vi "Init.vi"(8 "error in (no error)":errorcluster, 10 "Address":string, 11 "KIM101.lvlib:KIM101.lvclass":refnum<class "KIM101.lvclass">) -> (0 "error out":errorcluster, 3 "KIM101.lvlib:KIM101.lvclass":refnum<class "KIM101.lvclass">)   [LabVIEW 2023, in "KIM101.lvlib" / "KIM101.lvclass"]
uses:
  KIM101.lvclass
  C:/Program Files/National Instruments/LabVIEW 2023/vi.lib/ActorFramework/Actor/Actor.lvclass
  UIs/TranslationStage_UI/TranslationStage_UI/BPC_Voltages.ctl
  <vilib>/ActorFramework/Message Enqueuer/Message Enqueuer.lvclass
  typedefs/instrumentType.ctl
  KIM101.lvclass/KIM101.ctl
  <vilib>/ActorFramework/Actor/Actor.lvclass/Actor.ctl
  <vilib>/ActorFramework/Message Enqueuer/Message Enqueuer.lvclass/Message Enqueuer.ctl
  Interfaces/InitDeinitInterface/InitDeinitComm Messages/InitDone Msg/InitDone Msg.lvclass/InitDone Msg.ctl
  <vilib>/ActorFramework/Message Enqueuer/Init from Existing Queue.vi
  <vilib>/ActorFramework/Message Enqueuer/Enqueue.vi
  Interfaces/InitDeinitInterface/InitDeinitComm Messages/InitDone Msg/InitDone Msg.lvclass
  C:/Program Files/National Instruments/LabVIEW 2023/vi.lib/ActorFramework/Message/Message.lvclass
  <vilib>/ActorFramework/Message Priority Queue/Priority Enqueue.vi
  C:/Users/quantum/Documents/LVDAQ/UIs/TranslationStage_UI/Thorlabs.MotionControl.KCube.InertialMotorCLI.dll
  UIs/TranslationStage_UI/Thorlabs.MotionControl.KCube.InertialMotorCLI.dll
  KIM101.lvlib
  typedefs/typedefs.lvlib
  <vilib>/ActorFramework/Actor/Actor.lvclass
  C:/Users/quantum/Documents/LVDAQ/UIs/TranslationStage_UI/Thorlabs.MotionControl.Controls.dll
  UIs/TranslationStage_UI/Thorlabs.MotionControl.Controls.dll
panel:
  out "output cluster":T3
  out "KIM Enqueuer":refnum<class "Message Enqueuer.lvclass">
  in  "KIM Positions":T1
  in  "KCubeInertialMotorControl":refnum<k24>(container)
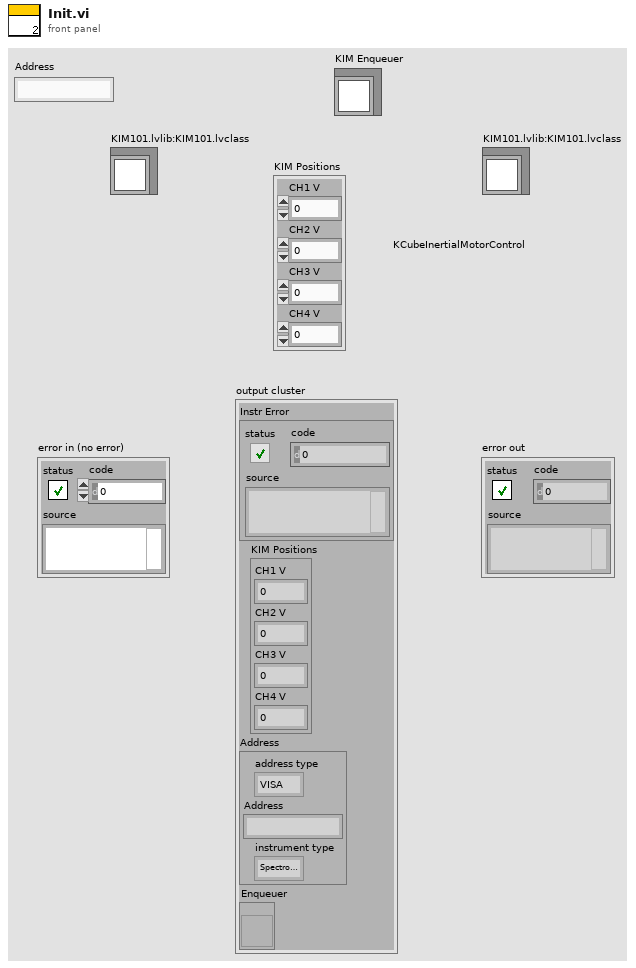
[diagram p1: front panel]
types:
  T1 = typedef "typedefs.lvlib/BPC_Voltages.ctl" = cluster{"CH1 V":i32, "CH2 V":i32, "CH3 V":i32, "CH4 V":i32}
  T2 = typedef "typedefs.lvlib/instrumentType.ctl" = enum16{"Spectrometer", "Camera", "Stepper", "Piezo"}
  T3 = cluster{"Instr Error":errorcluster, "KIM Positions":T1, "Address":cluster{"address type":enum16{"VISA", "Index"}, "Address":string, "instrument type":T2}, "Enqueuer":refnum<vi>}
  T4 = cluster{"JogAcceleration":i32, "JogStepFwd":i32, "JogMode":i32, "JogRate":i32, "JogStepRev":i32}
  T5 = cluster{"address type":enum16{"VISA", "Index"}, "Address":string, "instrument type":T2}
  T6 = cluster{"Instr Error":errorcluster, "KIM Positions":T1, "Address":cluster{"address type":enum16{"VISA", "Index"}, "Address":string, "instrument type":T2}, "KIM Enqueuer":refnum<vi>}
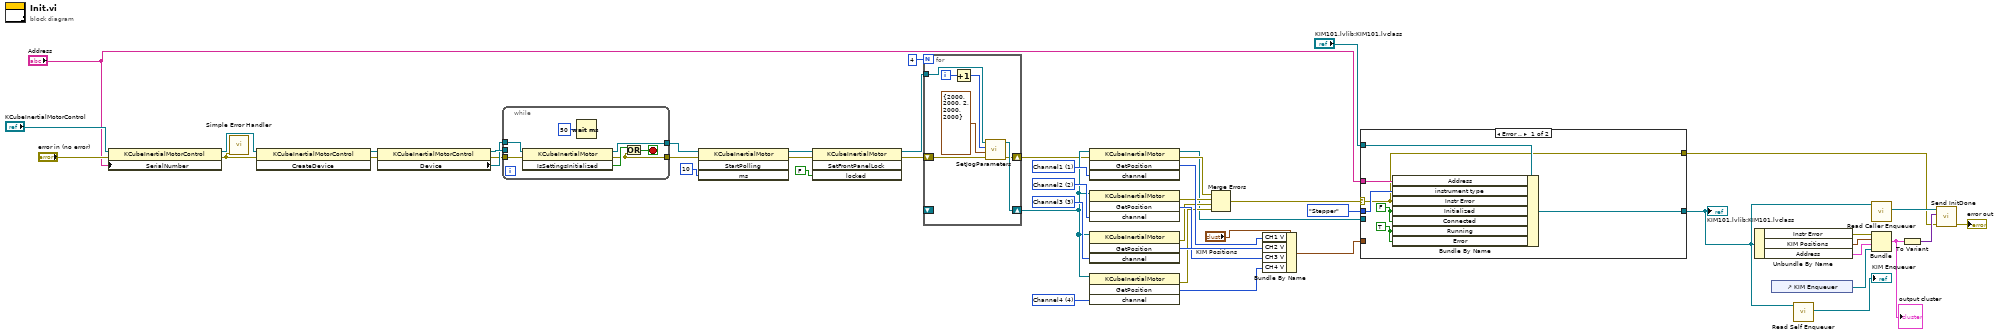
[diagram p0: block diagram]
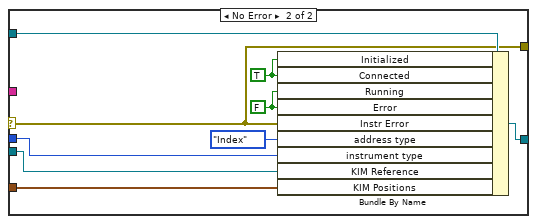
[diagram p2: hidden frame]
diagram:
  w34 = 4 items=["Channel1"=1, "Channel2"=2, "Channel3"=3, "Channel4"=4] ("channel")
  w35 = 3 items=["Channel1"=1, "Channel2"=2, "Channel3"=3, "Channel4"=4] ("channel")
  w36 = 2 items=["Channel1"=1, "Channel2"=2, "Channel3"=3, "Channel4"=4] ("channel")
  w37 = 1 items=["Channel1"=1, "Channel2"=2, "Channel3"=3, "Channel4"=4] ("channel")
  n1 = property class="KCubeInertialMotorControl"(reference="KCubeInertialMotorControl", error in="error in (no error)", "SerialNumber"="Address") -> (reference out=w40:refnum<k24>, error out=w38:errorcluster)
  n2 = call <vilib>:"Simple Error Handler.vi"("error in (no error)"=w38) -> ()  [unwired: 4 in, 5 out]
  n3 = invoke class="KCubeInertialMotorControl" method="CreateDevice"(reference=w40, error in=w38) -> (reference out=w47:refnum<k24>, error out=w48:errorcluster)  [unwired: 1 in, 1 out]
  n4 = property class="KCubeInertialMotorControl"(reference=w47, error in=w48) -> (reference out=w50:refnum<k24>, error out=w41:errorcluster, "Device"=w49:refnum<k24>)
  n5 = while {
    tunnel: w49 -> [w54]
    tunnel: [w57] -> w45
    tunnel: w41 -> [w55]
    tunnel: [w52] -> w44
    tunnel: w50 -> [_]
    stop <- w51 stop-if-true
    n6 = invoke class="KCubeInertialMotor" method="IsSettingsInitialized"(reference=w54, error in=w55) -> (reference out=w57:refnum<k24>, error out=w52:errorcluster, "IsSettingsInitialized"=w53:bool)  [unwired: 1 in]
    n7 = Wait (ms)(milliseconds to wait=u32 50) -> ()  [unwired: 1 out]
    n8 = Or(x=w53, y=w52) -> (x .or. y?=w51:bool)
  }
  n9 = invoke class="KCubeInertialMotor" method="StartPolling"(reference=w45, error in=w44, "ms"=10) -> (reference out=w20:refnum<k24>, error out=w18:errorcluster)  [unwired: 1 in, 2 out]
  n10 = invoke class="KCubeInertialMotor" method="SetFrontPanelLock"(reference=w20, error in=w18, "locked"=FALSE) -> (reference out=w16:refnum<k24>, error out=w17:errorcluster)  [unwired: 1 in, 2 out]
  n11 = for {
    N: 4 -> [_]
    tunnel: w16 -> [w63]
    shift-right: [w61] -> w14
    shift-left: w17 -> [w64]
    shift-right: [w62] -> w15
    shift-left: _ -> [_]
    i -> [w58]
    n12 = Increment(x=w58) -> (x+1=w59:i32)
    n13 = call "SetJogParameters.vi"("error in (no error)"=w64, "Jog Parameters"=T4 {"JogAcceleration"=2000, "JogStepFwd"=2000, "JogMode"=2, "JogRate"=2000, "JogStepRev"=2000} ("Jog Parameters 2"), "channel"=w59, "KIM Reference"=w63) -> ("error out"=w61:errorcluster, "KIM Reference"=w62:refnum<k24>)  [unwired: 6 in]
  }
  n14 = invoke class="KCubeInertialMotor" method="GetPosition"(reference=w15, error in=w14, "channel"=w37) -> (reference out=w22:refnum<k24>, error out=w28:errorcluster, "GetPosition"=w33:i32)  [unwired: 1 in, 1 out]
  n15 = invoke class="KCubeInertialMotor" method="GetPosition"(reference=w15, "channel"=w36) -> (error out=w29:errorcluster, "GetPosition"=w32:i32)  [unwired: 2 in, 2 out]
  n16 = invoke class="KCubeInertialMotor" method="GetPosition"(reference=w15, "channel"=w35) -> (error out=w27:errorcluster, "GetPosition"=w31:i32)  [unwired: 2 in, 2 out]
  n17 = invoke class="KCubeInertialMotor" method="GetPosition"(reference=w15, "channel"=w34) -> (error out=w26:errorcluster, "GetPosition"=w30:i32)  [unwired: 2 in, 2 out]
  n18 = Merge Errors(w28, w29, w27, w26) -> (w25:errorcluster)
  n19 = Bundle By Name(cluster="KIM Positions", "CH1 V"=w33, "CH2 V"=w32, "CH3 V"=w31, "CH4 V"=w30) -> (w11:T1)
  n20 = case shown="Error .." w25 {
    selector: w25 -> [w65 w72]
    tunnel: "KIM101.lvlib:KIM101.lvclass" -> [w66 w77]
    tunnel: [w67 w78] -> w5
    tunnel: instrumentType."Stepper" ("InstrumentData.Address.instrument type") -> [w71 w75]
    tunnel: "Address" -> [w70 _]
    tunnel: w22 -> [_ w73]
    tunnel: w11 -> [_ w74]
    tunnel: [w65 w72] -> w1
    frame Error {
      w68 = TRUE ("InstrumentData.CurrentState.Error")
      w69 = FALSE ("InstrumentData.CurrentState.Initialized")
      n21 = Bundle By Name(cluster=w66, "Address"=w70, "instrument type"=w71, "Instr Error"=w65, "Initialized"=w69, "Connected"=w69, "Running"=w68, "Error"=w68) -> (w67:refnum<class "KIM101.lvclass">)
    }
    frame No Error {
      w79 = FALSE ("InstrumentData.CurrentState.Error")
      w80 = TRUE ("InstrumentData.CurrentState.Initialized")
      n22 = Bundle By Name(cluster=w77, "Initialized"=w80, "Connected"=w80, "Running"=w79, "Error"=w79, "Instr Error"=w72, "address type"=enum16{"VISA", "Index"}."Index" ("InstrumentData.Address.address type"), "instrument type"=w75, "KIM Reference"=w73, "KIM Positions"=w74) -> (w78:refnum<class "KIM101.lvclass">)
    }
  }
  "KIM101.lvlib:KIM101.lvclass" <- w5
  n23 = Unbundle By Name(w5) -> ("Instr Error"=w10:errorcluster, "KIM Positions"=w9:T1, "Address"=w8:T5)
  n24 = control-ref of="KIM Enqueuer"() -> (w3:refnum<vi>)
  n25 = call <vilib>:"Read Self Enqueuer.vi"("Actor"=w5) -> ("Self Enqueuer"=→"KIM Enqueuer":refnum<class "Message Enqueuer.lvclass">)  [unwired: 10 in]
  n26 = call <vilib>:"Read Caller Enqueuer.vi"("Actor"=w5) -> ("Caller Enqueuer"=w24:refnum<class "Message Enqueuer.lvclass">)  [unwired: 10 in]
  n27 = Bundle("Instr Error"=w10, "KIM Positions"=w9, "Address"=w8, "KIM Enqueuer"=w3) -> (w7:T6)  [unwired: 1 in]
  "output cluster" <- w7
  n28 = To Variant(anything=w7) -> (Variant=w6:variant)
  n29 = call "Send InitDone.vi"("error in (no error)"=w1, "Variant"=w6, "Message Enqueuer"=w24) -> ("error out"=→"error out":errorcluster)  [unwired: 7 in, 1 out]
